vi "Test Registration Event to JSON.vi"(9 "indent level":i32, 10 "Test Registration":T1) -> (2 "<JSON>Test Registration Event":string)   [LabVIEW 2013, in "Caraya.lvlib" / "Test Result.lvclass"]
uses:
  Test Result.lvclass
  Test Registration Data.ctl
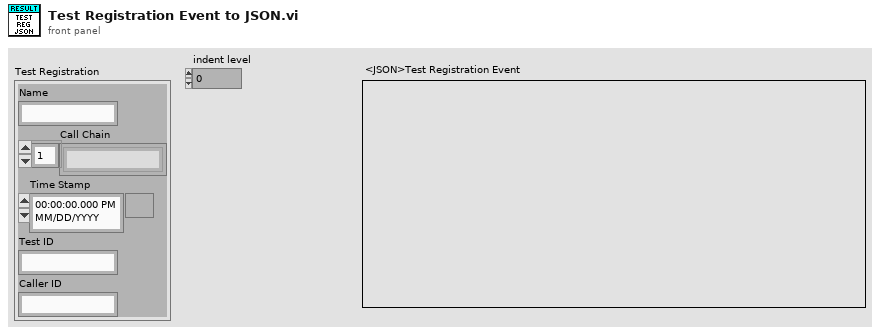
[diagram p1: front panel]
types:
  T1 = typedef "Caraya.lvlib/Test Result.lvclass/Test Registration Data.ctl" = cluster{"Name":string, "Call Chain":string[], "Time Stamp":timestamp, "Test ID":string, "Caller ID":string}
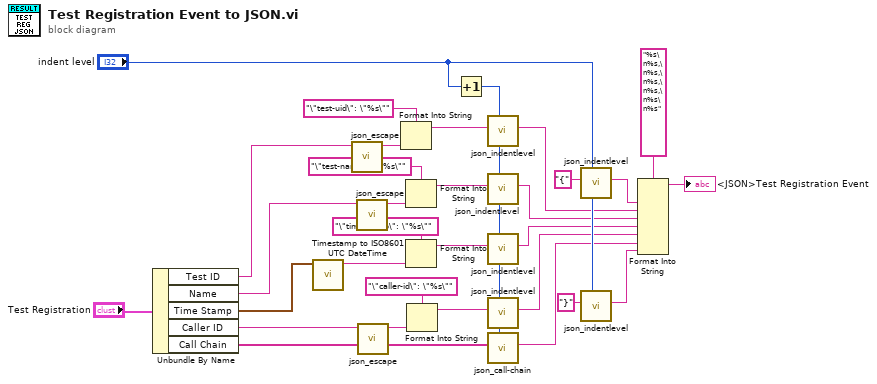
[diagram p0: block diagram]
diagram:
  n1 = Unbundle By Name("Test Registration") -> ("Test ID"=w21:string, "Name"=w13:string, "Time Stamp"=w12:timestamp, "Caller ID"=w14:string, "Call Chain"=w3:string[])
  n2 = call <vilib>:"Timestamp to ISO8601 UTC DateTime.vi"("Timestamp (now)"=w12) -> ("ISO8601 UTC DateTime"=w11:string)  [unwired: 10 in]
  n3 = call "json_escape.vi"("string"=w21) -> ("escaped string"=w23:string)  [unwired: 10 in]
  n4 = call "json_escape.vi"("string"=w13) -> ("escaped string"=w19:string)  [unwired: 10 in]
  n5 = call "json_escape.vi"("string"=w14) -> ("escaped string"=w16:string)  [unwired: 10 in]
  n6 = Format Into String(format string="\"test-uid\": \"%s\"", w23) -> (resulting string=w26:string)  [unwired: 2 in, 1 out]
  n7 = Format Into String(format string="\"test-name\": \"%s\"", w19) -> (resulting string=w4:string)  [unwired: 2 in, 1 out]
  n8 = Format Into String(format string="\"timestamp\": \"%s\"", w11) -> (resulting string=w5:string)  [unwired: 2 in, 1 out]
  n9 = Format Into String(format string="\"caller-id\": \"%s\"", w16) -> (resulting string=w6:string)  [unwired: 2 in, 1 out]
  n10 = Increment(x="indent level") -> (x+1=w2:i32)
  n11 = call "json_indentlevel.vi"("indent level"=w2, "string"=w26) -> ("indented string"=w24:string)  [unwired: 9 in]
  n12 = call "json_indentlevel.vi"("indent level"=w2, "string"=w4) -> ("indented string"=w10:string)  [unwired: 9 in]
  n13 = call "json_indentlevel.vi"("indent level"=w2, "string"=w5) -> ("indented string"=w9:string)  [unwired: 9 in]
  n14 = call "json_indentlevel.vi"("indent level"=w2, "string"=w6) -> ("indented string"=w8:string)  [unwired: 9 in]
  n15 = call "json_call-chain.vi"("indent level"=w2, "Call Chain"=w3) -> ("indented string"=w1:string)  [unwired: 9 in]
  n16 = call "json_indentlevel.vi"("indent level"="indent level", "string"="{") -> ("indented string"=w29:string)  [unwired: 9 in]
  n17 = call "json_indentlevel.vi"("indent level"="indent level", "string"="}") -> ("indented string"=w7:string)  [unwired: 9 in]
  n18 = Format Into String(format string="%s\n%s,\n%s,\n%s,\n%s,\n%s\n%s", w29, w24, w10, w9, w8, w1, w7) -> (resulting string=→"<JSON>Test Registration Event":string)  [unwired: 2 in, 1 out]
